vi "4.5.vi"(1 "指定值":dbl) -> (0 "循环次数":i32, 2 "随机数":dbl)   [LabVIEW 2017]
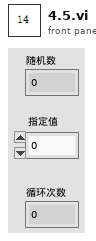
[diagram p1: front panel]
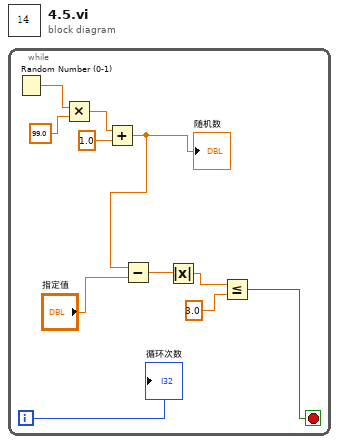
[diagram p0: block diagram]
diagram:
  n1 = while {
    i -> [w5]
    stop <- w6 stop-if-true
    n2 = Random Number (0-1)() -> (number: 0 to 1=w4:dbl)
    n3 = Multiply(x=w4, y=99.0) -> (x*y=w3:dbl)
    n4 = Add(x=w3, y=1.0) -> (x+y=w1:dbl)
    "随机数" <- w1
    n5 = Subtract(x=w1, y="指定值") -> (x-y=w9:dbl)
    n6 = Absolute Value(x=w9) -> (abs(x)=w8:dbl)
    n7 = Less Or Equal?(x=w8, y=3.0) -> (x <= y?=w6:bool)
    "循环次数" <- w5
  }
